vi "Update Channel Name.vi"(5 "Display State In":T1={"Current Channels Info"=[], "Help Prefix"="", "Max Display Size"=8, "Max Size"=8, "Show Buttons"=TRUE, "Data Valid"=refnum, "Show Range"=FALSE, "Range Items"=[], "Range Index"=[]} caption="State", 8 "error in (no error)":errorcluster, 11 "Channel Name Reference":refnum<vi>) -> (0 "error out":errorcluster)   [LabVIEW 2021, in "myRIO Channel List.xctl"]
uses:
  <vilib>/myRIO/Common/Express VI Framework/xctls/myRIO Channel List/myRIO Channel List.xctl
  <vilib>/myRIO/Common/Express VI Framework/xctls/myRIO Channel List/State.ctl
  <vilib>/myRIO/Common/Profile Manager Framework/typedefs/Channel Info.ctl
  <vilib>/myRIO/Common/Express VI Framework/typedefs/Data Validate Ref.ctl
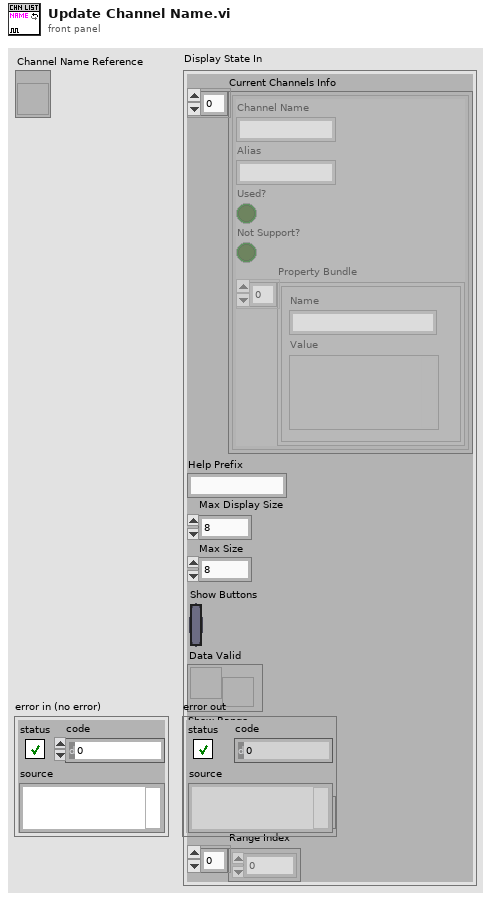
[diagram p1: front panel]
types:
  T1 = typedef "myRIO Channel List.xctl/State.ctl" = cluster{"Current Channels Info":T2[], "Help Prefix":string, "Max Display Size":i32, "Max Size":i32, "Show Buttons":bool, "Data Valid":T3, "Show Range":bool, "Range Items":string[], "Range Index":i32[]}
  T2 = typedef "Channel Info.ctl" = cluster{"Channel Name":string, "Alias":string, "Used?":bool, "Not Support?":bool, "Property Bundle":cluster{"Name":string, "Value":variant}[]}
  T3 = typedef "Data Validate Ref.ctl" = refnum<user-event>
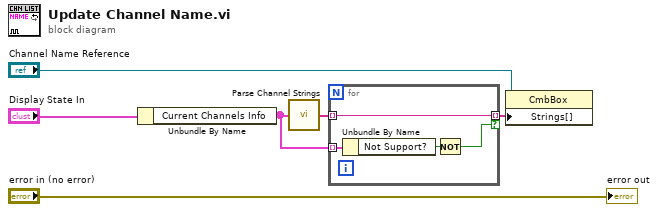
[diagram p0: block diagram]
diagram:
  n1 = Unbundle By Name("Display State In") -> ("Current Channels Info"=w2:T2[])
  n2 = call <vilib>:"Parse Channel Strings.vi"("Channels Info"=w2) -> ("Channel Strings"=w3:string[])
  n3 = for {
    tunnel: w3 -> [w10] mode=indexing
    tunnel: [w10] -> w1 mode=indexing if=w7
    tunnel: w2 -> [w9] mode=indexing
    n4 = Unbundle By Name(w9) -> ("Not Support?"=w8:bool)
    n5 = Not(x=w8) -> (.not. x?=w7:bool)
  }
  n6 = property class="CmbBox"(reference="Channel Name Reference", "Strings[]"=w1) -> ()  [unwired: 1 in, 2 out]
  "error out" <- "error in (no error)"
